vi "compsInit.vi"(1 "XY stage":T1, 2 "Filter wheel init":cluster{"FW Handle":u32, "init?":i16}, 3 "sCMOS init":cluster{"init":i16, "sCMOS handle":u32}, 4 "Z stage":T2) -> (0 "allComponentsInit?":bool)   [LabVIEW 2015]
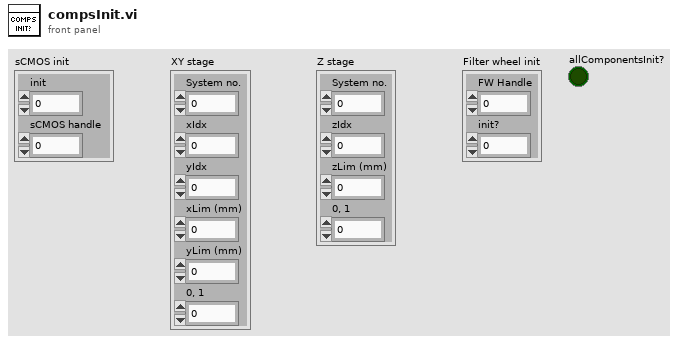
[diagram p1: front panel]
types:
  T1 = cluster{"System no.":i32, "xIdx":i32, "yIdx":i32, "xLim (mm)":dbl, "yLim (mm)":dbl, "0, 1":i16}
  T2 = cluster{"System no.":i32, "zIdx":i32, "zLim (mm)":dbl, "0, 1":i16}
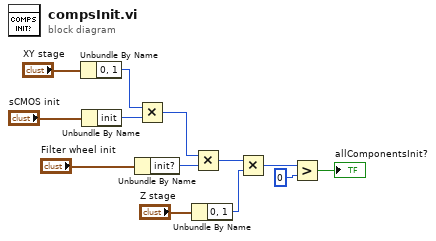
[diagram p0: block diagram]
diagram:
  n1 = Unbundle By Name("XY stage") -> ("0, 1"=w6:i16)
  n2 = Unbundle By Name("sCMOS init") -> ("init"=w7:i16)
  n3 = Unbundle By Name("Filter wheel init") -> ("init?"=w9:i16)
  n4 = Multiply(x=w6, y=w7) -> (x*y=w8:i16)
  n5 = Unbundle By Name("Z stage") -> ("0, 1"=w11:i16)
  n6 = Multiply(x=w8, y=w9) -> (x*y=w10:i16)
  n7 = Multiply(x=w10, y=w11) -> (x*y=w13:i16)
  n8 = Greater?(x=w13, y=0) -> (0:→"allComponentsInit?":bool)
